vi "Teleop.vi"(10 "Match Info":T1={"Autonomous Elapsed Seconds"=0.0, "TeleOp Elapsed Seconds"=0.0, "Disabled Elapsed Seconds"=0.0, "Visited Autonomous"=FALSE, "Visited TeleOp"=FALSE, "Visited Disabled"=FALSE, "Autonomous Settings"={"Autonomous Style"=enum."Independent", "VI Refnum"=refnum}}, 11 "Call Context":T2) -> ()   [LabVIEW 2013]
doc: "This VI is called for each TeleOp packet received from the DS where the robot is not disabled. It is often used to read from the joysticks and update I/O or to update setpoints for timed control loops. It should complete and return within 20 milliseconds or it may miss DS packets."
uses:
  <vilib>/Rock Robotics/WPI/DriverStation/WPI_DriverStationDerivedRobotMode.ctl
  <vilib>/Rock Robotics/WPI/DriverStation/WPI_DriverStationMatch Info.ctl
  Robot Global Data.vi
  <vilib>/Rock Robotics/WPI/Joystick/WPI_JoystickGetSetRefNum.vi
  <vilib>/Rock Robotics/WPI/RobotDrive/WPI_RobotDriveGetSetRefNum.vi
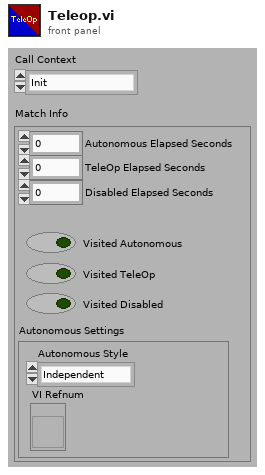
[diagram p1: front panel]
types:
  T1 = typedef "WPI_DriverStationMatch Info.ctl" = cluster{"Autonomous Elapsed Seconds":dbl, "TeleOp Elapsed Seconds":dbl, "Disabled Elapsed Seconds":dbl, "Visited Autonomous":bool, "Visited TeleOp":bool, "Visited Disabled":bool, "Autonomous Settings":cluster{"Autonomous Style":enum16{"Iterative", "Independent"}, "VI Refnum":refnum<vi>}}
  T2 = typedef "WPI_DriverStationDerivedRobotMode.ctl" = enum16{"Init", "Execute", "Stop"}
  T3 = typedef "WPI_JoystickDevRef.ctl" = cluster{"Device":T4}
  T4 = typedef "WPI_JoystickDeviceEnum.ctl" = enum16{"USB 1", "USB 2", "USB 3", "USB 4", "Kinect 1", "Kinect 2"}
  T5 = typedef "WPI_JoystickButtonState.ctl" = cluster{"Button 1":bool, "Button 2":bool, "Button 3":bool, "Button 4":bool, "Button 5":bool, "Button 6":bool, "Button 7":bool, "Button 8":bool, "Button 9":bool, "Button 10":bool, "Button 11":bool, "Button 12":bool}
  T6 = cluster{"axis 1 (x)":dbl, "axis 2 (y)":dbl, "axis 3 (throttle)":dbl, "axis 4":dbl, "axis 5":dbl, "axis 6":dbl}
  T7 = typedef "WPI_RobotDriveDevRef.ctl" = cluster{"DevStatus":errorcluster, "Motors[]":T8[], "Square Inputs":bool, "Max Output":dbl, "Isochronous":bool}
  T8 = typedef "WPI_MotorControlDeviceRef.ctl" = cluster{"DeviceStatus":errorcluster, "Type":enum16{"PWM", "CAN"}, "PWM":cluster{"Digital Module":T9, "PWM Channel":T10, "DeadBand":T11}, "CAN":cluster{"Device Number":u8, "Control Mode":T12, "Semaphore":T13, "Max Vout":dbl}, "Invert":bool, "TransformRef":T14, "InvTransformRef":T14}
  T9 = typedef "FPGA_TypedefDigitalModule.ctl" = enum16{"Digital Module 1", "Digital Module 2"}
  T10 = typedef "FPGA_DIOPWMChannel.ctl" = enum8{"PWM 1", "PWM 2", "PWM 3", "PWM 4", "PWM 5", "PWM 6", "PWM 7", "PWM 8", "PWM 9", "PWM 10", "Invalid"}
  T11 = typedef "WPI_PWMDeadband.ctl" = cluster{"Name":string, "maxPositivePwm":i32, "minPositivePwm":i32, "centerPwm":i32, "maxNegativePwm":i32, "minNegativePwm":i32, "angularRange":u16}
  T12 = typedef "WPI_CANJaguar_ControlMode.ctl" = enum8{"Percent VBus", "Current", "Speed", "Position", "Voltage"}
  T13 = typedef "Semaphore RefNum" = refnum<k1>
  T14 = typedef "WPI_PWMTransform_ConPane.ctl" = refnum<vi>
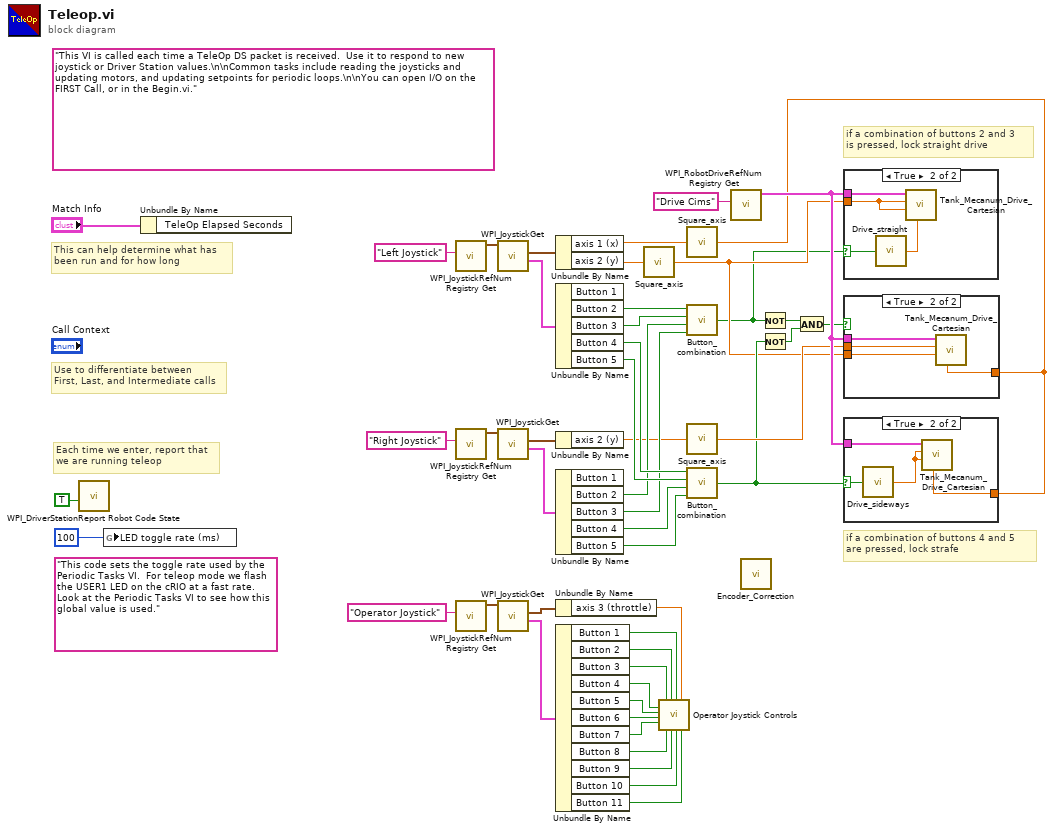
[diagram p0: block diagram]
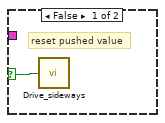
[diagram p3: hidden frame]
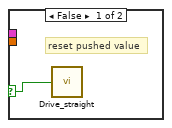
[diagram p4: hidden frame]
diagram:
  (unwired) "This code sets the toggle rate used by the Periodic Tasks VI.  For teleop mode we flash the USER1 LED on the cRIO at a fast rate.  Look at the Periodic Tasks VI to see how this global value is used."
  (unwired) "This VI is called each time a TeleOp DS packet is received.  Use it to respond to new joystick or Driver Station values.\n\nCommon tasks include reading the joysticks and updating motors, and updating setpoints for periodic loops.\n\nYou can open I/O on the FIRST Call, or in the Begin.vi."
  # "if a combination of buttons 2 and 3\nis pressed, lock straight drive"
  # "if a combination of buttons 4 and 5 \nare pressed, lock strafe"
  # "Each time we enter, report that\nwe are running teleop"
  # "Use to differentiate between\nFirst, Last, and Intermediate calls"
  # "This can help determine what has\nbeen run and for how long"
  n1 = call <vilib>:"WPI_DriverStationReport Robot Code State.vi"("TeleOp"=TRUE ("Autonomous")) -> ()  [unwired: 10 in, 1 out]
  n2 = global write "Robot Global Data.vi" "LED toggle rate (ms)"(u32 100 ("LED ms toggle rate")) -> ()
  n3 = Unbundle By Name("Match Info") -> ()  [unwired: 1 out]
  n4 = call <vilib>:"WPI_JoystickRefNum Registry Get.vi"("refnum name"="Left Joystick") -> ("JoystickDevRef"=w41:T3)  [unwired: 9 in, 1 out]
  n5 = call <vilib>:"WPI_JoystickRefNum Registry Get.vi"("refnum name"="Right Joystick") -> ("JoystickDevRef"=w42:T3)  [unwired: 9 in, 1 out]
  n6 = call <vilib>:"WPI_JoystickRefNum Registry Get.vi"("refnum name"="Operator Joystick") -> ("JoystickDevRef"=w38:T3)  [unwired: 9 in, 1 out]
  n7 = call <vilib>:"WPI_JoystickGet.vi"("JoystickDevRef"=w41) -> ("Buttons"=w22:T5, "Axes"=w40:T6)  [unwired: 4 in, 1 out]
  n8 = call <vilib>:"WPI_JoystickGet.vi"("JoystickDevRef"=w42) -> ("Buttons"=w23:T5, "Axes"=w36:T6)  [unwired: 4 in, 1 out]
  n9 = call <vilib>:"WPI_JoystickGet.vi"("JoystickDevRef"=w38) -> ("Buttons"=w1:T5, "Axes"=w37:T6)  [unwired: 4 in, 1 out]
  n10 = Unbundle By Name(w40) -> ("axis 1 (x)"=w14:dbl, "axis 2 (y)"=w19:dbl)
  n11 = Unbundle By Name(w22) -> ("Button 2"=w18:bool, "Button 3"=w13:bool, "Button 4"=w17:bool, "Button 5"=w16:bool)  [unwired: 1 out]
  n12 = Unbundle By Name(w36) -> ("axis 2 (y)"=w10:dbl)
  n13 = Unbundle By Name(w23) -> ("Button 2"=w12:bool, "Button 3"=w11:bool, "Button 4"=w15:bool, "Button 5"=w9:bool)  [unwired: 1 out]
  n14 = Unbundle By Name(w37) -> ("axis 3 (throttle)"=w35:dbl)
  n15 = Unbundle By Name(w1) -> ("Button 1"=w34:bool, "Button 2"=w33:bool, "Button 3"=w32:bool, "Button 4"=w31:bool, "Button 5"=w30:bool, "Button 6"=w29:bool, "Button 7"=w28:bool, "Button 8"=w27:bool, "Button 9"=w26:bool, "Button 10"=w25:bool, "Button 11"=w24:bool)
  n16 = call "Square_axis.vi"("axis"=w19) -> ("axis squared"=w3:dbl)
  n17 = call "Operator Joystick Controls.vi"("Button 4"=w31, "Button 5"=w30, "Button 6"=w29, "Button 7"=w28, "Button 3"=w32, "Button 8"=w27, "Button 2"=w33, "Button 9"=w26, "Button 1"=w34, "Button 10"=w25, "axis 3 (throttle)"=w35, "Button 11"=w24) -> ()  [unwired: 8 in]
  n18 = call "Square_axis.vi"("axis"=w14) -> ("axis squared"=w7:dbl)
  n19 = call "Button_combination.vi"("Right 2"=w11, "Right 1"=w12, "Left 2"=w13, "Left 1"=w18) -> ("Combination"=w2:bool)
  n20 = call "Square_axis.vi"("axis"=w10) -> ("axis squared"=w5:dbl)
  n21 = call "Button_combination.vi"("Right 2"=w9, "Right 1"=w15, "Left 2"=w16, "Left 1"=w17) -> ("Combination"=w4:bool)
  n22 = call <vilib>:"WPI_RobotDriveRefNum Registry Get.vi"("refnum name"="Drive Cims") -> ("RobotDriveDevRef"=w8:T7)  [unwired: 9 in, 1 out]
  n23 = call "Encoder_Correction.vi"() -> ()  [unwired: 12 in]
  n24 = Not(x=w2) -> (.not. x?=w21:bool)
  n25 = Not(x=w4) -> (.not. x?=w20:bool)
  n26 = And(x=w21, y=w20) -> (x .and. y?=w6:bool)
  n27 = case shown="True" w2 {
    selector: w2 -> [w49 w51]
    tunnel: w8 -> [_ w53]
    tunnel: w3 -> [_ w52]
    frame False {
      # "reset pushed value"
      n28 = call "Drive_straight.vi"("Buttons pushed?"=w49) -> ()  [unwired: 3 in, 2 out]
    }
    frame True {
      n29 = call "Drive_straight.vi"("Buttons pushed?"=w51) -> ("output"=w50:dbl)  [unwired: 3 in, 1 out]
      n30 = call "Tank_Mecanum_Drive_Cartesian.vi"("Left X"=w50, "Left Y"=w52, "Right Y"=w52, "RobotDriveDevRef"=w53) -> ()  [unwired: 5 in, 3 out]
    }
  }
  n31 = case shown="True" w6 {
    tunnel: w8 -> [_ w57]
    tunnel: w3 -> [_ w56]
    tunnel: w5 -> [_ w55]
    tunnel: w7 -> [_ w54]
    frame False {
    }
    frame True {
      n32 = call "Tank_Mecanum_Drive_Cartesian.vi"("Left X"=w54, "Left Y"=w56, "Right Y"=w55, "RobotDriveDevRef"=w57) -> ()  [unwired: 5 in, 3 out]
    }
  }
  n33 = case shown="True" w4 {
    selector: w4 -> [w58 w61]
    tunnel: w8 -> [_ w62]
    tunnel: w7 -> [_ w60]
    frame False {
      # "reset pushed value"
      n34 = call "Drive_sideways.vi"("Buttons pushed?"=w58) -> ()  [unwired: 3 in, 2 out]
    }
    frame True {
      n35 = call "Drive_sideways.vi"("Buttons pushed?"=w61) -> ("output"=w59:dbl)  [unwired: 3 in, 1 out]
      n36 = call "Tank_Mecanum_Drive_Cartesian.vi"("Left X"=w60, "Left Y"=w59, "Right Y"=w59, "RobotDriveDevRef"=w62) -> ()  [unwired: 5 in, 3 out]
    }
  }
